vi "Write TDMS.vi"(8 "error in":errorcluster, 11 "Control Loop Cluster":T1) -> (0 "error out":errorcluster, 3 "Control Loop Cluster Out":T1)   [LabVIEW 2019, in "RT Main.lvlib"]
uses:
  RT Main.lvlib
  Control Loop Cluster.ctl
  <vilib>/myRIO/Instrument Drivers/Onboard IO/AI/typedefs/AI Reference.ctl
  <vilib>/myRIO/Common/Instrument Driver Framework/Utilities/typedefs/myRIO Generic Hardware Reference.ctl
  <vilib>/myRIO/Common/Instrument Driver Framework/Utilities/typedefs/Hardware Version Enum.ctl
  <vilib>/myRIO/Common/Instrument Driver Framework/Utilities/typedefs/myRIO v1.0 Reference.ctl
  <vilib>/myRIO/Common/Instrument Driver Framework/Utilities/typedefs/Generic FPGA Reference.ctl
  <vilib>/myRIO/Common/Instrument Driver Framework/myRIO v1.0/AI/typedefs/AI Channels List.ctl
  <vilib>/myRIO/Common/Instrument Driver Framework/myRIO v1.0/AI/typedefs/AI Channels Enum.ctl
  <vilib>/myRIO/Common/Instrument Driver Framework/Utilities/typedefs/Analog Scaling Constants List.ctl
  <vilib>/myRIO/Common/Instrument Driver Framework/Utilities/typedefs/Analog Scaling Constants.ctl
  <vilib>/myRIO/Instrument Drivers/Onboard IO/DIO/typedefs/DIO Reference.ctl
  <vilib>/myRIO/Common/Instrument Driver Framework/myRIO v1.0/DIO/typedefs/DIO Channels List.ctl
  <vilib>/myRIO/Common/Instrument Driver Framework/myRIO v1.0/DIO/typedefs/DIO Channels Enum.ctl
  Data Cluster.ctl
  Hardware Monitoring.ctl
  Modules/TDMS/TDMS.lvlib
  <vilib>/myRIO/Instrument Drivers/Onboard IO/AI/AI.lvlib
  <vilib>/myRIO/Instrument Drivers/Onboard IO/DIO/DIO.lvlib
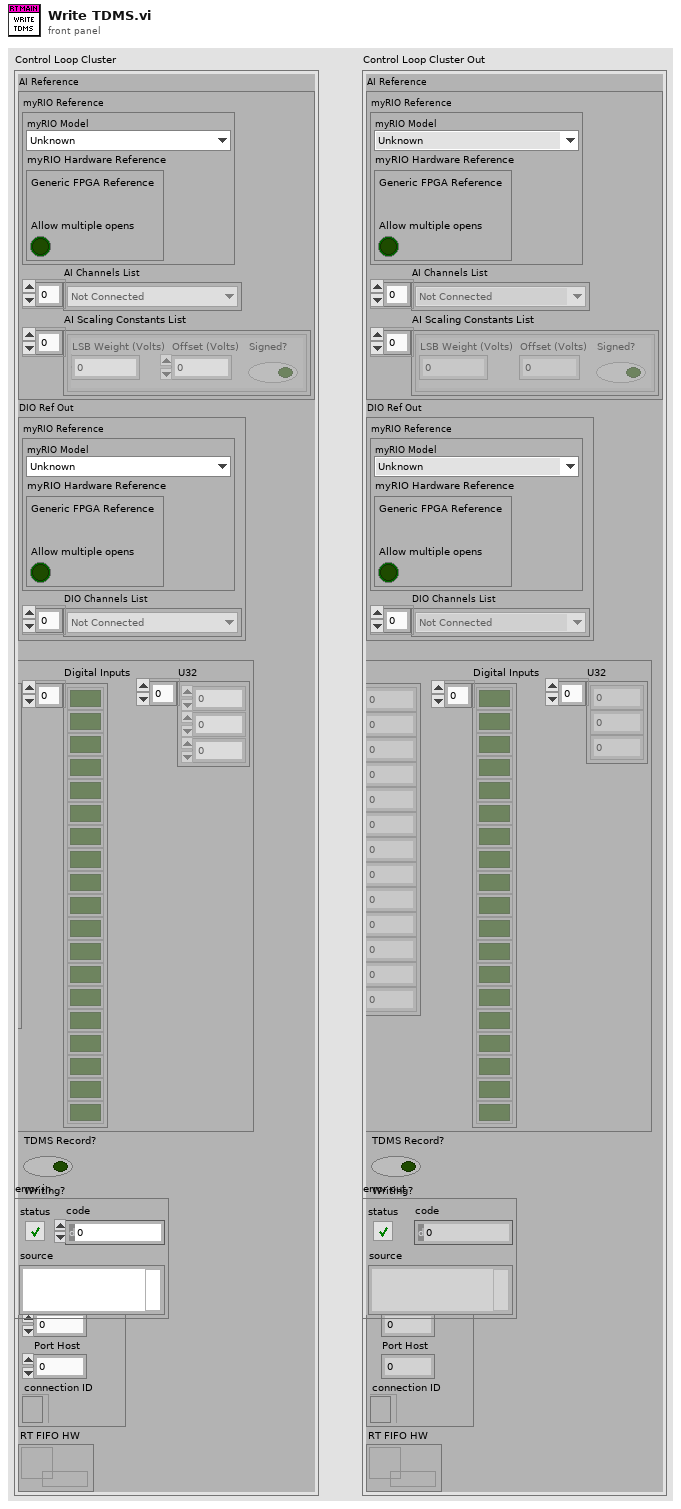
[diagram p1: front panel]
types:
  T1 = typedef "RT Main.lvlib/Control Loop Cluster.ctl" = cluster{"AI Reference":T2, "DIO Reference":T11, "Data Cluster":T14, "TDMS Record?":bool, "Writing?":bool, "UDP Info":cluster{"IP Host":string, "Port RT":u16, "Port Host":u16, "connection ID":refnum<k16>}, "RT FIFO HW":refnum<k33>}
  T2 = typedef "AI.lvlib/AI Reference.ctl" = cluster{"myRIO Reference":T3, "AI Channels List":T7, "AI Scaling Constants List":T9}
  T3 = typedef "myRIO Generic Hardware Reference.ctl" = cluster{"myRIO Model":T4, "myRIO Hardware Reference":T5}
  T4 = typedef "Hardware Version Enum.ctl" = enum16{"Unknown", "myRIO-1900", "myRIO-1950", "roboRIO", "NI ELVIS RIO CM", "ELVIS III"}
  T5 = typedef "myRIO v1.0 Reference.ctl" = cluster{"Generic FPGA Reference":T6, "Allow multiple opens":bool}
  T6 = typedef "Generic FPGA Reference.ctl" = refnum<k20>
  T7 = typedef "AI Channels List.ctl" = T8[]
  T8 = typedef "AI Channels Enum.ctl" = enum16{"Not Connected", "AudioIn/Left", "AudioIn/Right", "C/AI0", "C/AI1", "A/AI0", "A/AI1", "A/AI2", "A/AI3", "A/AI4", "A/AI5", "A/AI6", "A/AI7", "B/AI0", "B/AI1", "B/AI2", "B/AI3", "B/AI4", "B/AI5", "B/AI6", "B/AI7", "AI/AI0", "AI/AI1", "AI/AI2", "AI/AI3", "A/AI0 (DIFF)", "A/AI1 (DIFF)", "A/AI2 (DIFF)", "A/AI3 (DIFF)", "B/AI0 (DIFF)", "B/AI1 (DIFF)", "B/AI2 (DIFF)", "B/AI3 (DIFF)"}
  T9 = typedef "Analog Scaling Constants List.ctl" = T10[]
  T10 = typedef "Analog Scaling Constants.ctl" = cluster{"LSB Weight (Volts)":dbl, "Offset (Volts)":dbl, "Signed?":bool}
  T11 = typedef "DIO.lvlib/DIO Reference.ctl" = cluster{"myRIO Reference":T3, "DIO Channels List":T12}
  T12 = typedef "DIO Channels List.ctl" = T13[]
  T13 = typedef "DIO Channels Enum.ctl" = enum16{"Not Connected", "C/DIO0", "C/DIO1", "C/DIO2", "C/DIO3", "C/DIO4", "C/DIO5", "C/DIO6", "C/DIO7", "A/DIO0", "A/DIO1", "A/DIO2", "A/DIO3", "A/DIO4", "A/DIO5", "A/DIO6", "A/DIO7", "A/DIO8", "A/DIO9", "A/DIO10", "A/DIO11", "A/DIO12", "A/DIO13", "A/DIO14", "A/DIO15", "A/DIO16", "A/DIO17", "A/DIO18", "A/DIO19", "B/DIO0", "B/DIO1", "B/DIO2", "B/DIO3", "B/DIO4", "B/DIO5", "B/DIO6", "B/DIO7", "B/DIO8", "B/DIO9", "B/DIO10", "B/DIO11", "B/DIO12", "B/DIO13", "B/DIO14", "B/DIO15", "B/DIO16", "B/DIO17", "B/DIO18", "B/DIO19", "LED0", "LED1", "LED2", "LED3", "Button0", "DIO/DIO0", "DIO/DIO1", "DIO/DIO2", "DIO/DIO3", "DIO/DIO4", "DIO/DIO5", "DIO/DIO6", "DIO/DIO7", "DIO/DIO8", "DIO/DIO9", "SPI/CS0", "SPI/CS1", "SPI/CS2", "SPI/CS3", "LED RADIO (Green)", "LED RADIO (Red)", "LED COMM (Green)", "LED COMM (Red)", "LED MODE (Green)", "LED MODE (Red)"}
  T14 = typedef "RT Main.lvlib/Data Cluster.ctl" = cluster{"Analog Input":dbl[], "Digital Inputs":bool[], "U32":u32[]}
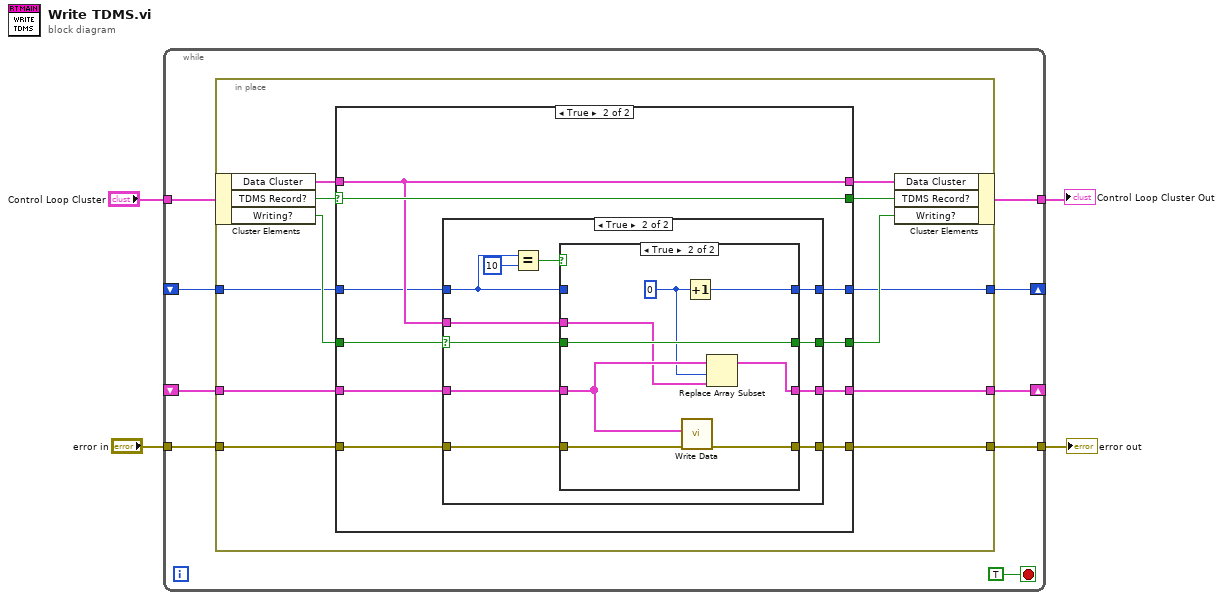
[diagram p0: block diagram]
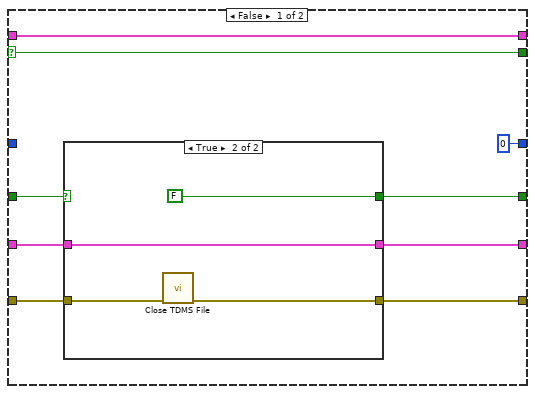
[diagram p2: hidden frame]
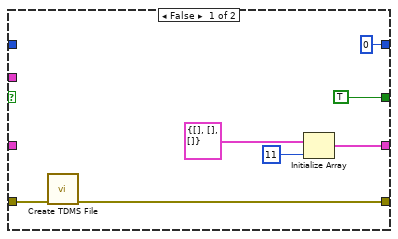
[diagram p4: hidden frame]
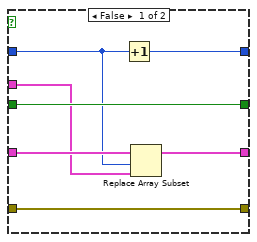
[diagram p5: hidden frame]
diagram:
  n1 = while {
    tunnel: "Control Loop Cluster" -> [w13]
    tunnel: "error in" -> [w12]
    tunnel: [w11] -> w2
    tunnel: [w9] -> w1
    shift-right: [w8] -> _
    shift-left: _ -> [w7]
    shift-right: [w6] -> _
    shift-left: _ -> [w5]
    stop <- TRUE stop-if-true
    n2 = in-place {
      in-place-border: w12 -> [w21]
      in-place-border: [w20] -> w9
      in-place-border: [w19] -> w8
      in-place-border: w7 -> [w18]
      in-place-border: [w15] -> w6
      in-place-border: w5 -> [w14]
      n3 = in-place-cluster #1(w13) -> ("Data Cluster"=w22:T14, "TDMS Record?"=w25:bool, "Writing?"=w17:bool)
      n4 = case shown="True" w25 {
        selector: w25 -> [w34 w51]
        tunnel: [w34 w51] -> w24
        tunnel: [w33 w46] -> w23
        tunnel: w22 -> [w33 w46]
        tunnel: [w31 w50] -> w16
        tunnel: w17 -> [w32 w49]
        tunnel: w21 -> [w30 w48]
        tunnel: [w29 w47] -> w20
        tunnel: [w27 w45] -> w19
        tunnel: w18 -> [w26 w44]
        tunnel: [0 w43] -> w15
        tunnel: w14 -> [_ w42]
        frame False {
          n5 = case shown="True" w32 {
            selector: w32 -> [w37 _]
            tunnel: [w37 FALSE] -> w31
            tunnel: w30 -> [w36 w40]
            tunnel: [w36 w39] -> w29
            tunnel: [w35 w38] -> w27
            tunnel: w26 -> [w35 w38]
            frame False {
            }
            frame True {
              n6 = call "Close TDMS File.vi"("error in"=w40) -> ("error out"=w39:errorcluster)  [unwired: 10 in]
            }
          }
        }
        frame True {
          n7 = case shown="True" w49 {
            selector: w49 -> [_ w68]
            tunnel: [TRUE w69] -> w50
            tunnel: w48 -> [w57 w67]
            tunnel: [w56 w66] -> w47
            tunnel: w46 -> [_ w65]
            tunnel: [w54 w63] -> w45
            tunnel: w44 -> [_ w64]
            tunnel: [0 w62] -> w43
            tunnel: w42 -> [_ w59]
            frame False {
              n8 = call "Create TDMS File.vi"("error in"=w57) -> ("error out"=w56:errorcluster)  [unwired: 10 in]
              n9 = Initialize Array(T14 {"Analog Input"=[], "Digital Inputs"=[], "U32"=[]} ("Data Cluster"), 11 ("dimension size")) -> (w54:T14[])
            }
            frame True {
              n10 = Equal?(x=w59, y=10) -> (x = y?=w61:bool)
              n11 = case shown="True" w61 {
                tunnel: [w76 w84] -> w69
                tunnel: w68 -> [w76 w84]
                tunnel: w67 -> [w75 w83]
                tunnel: [w75 w82] -> w66
                tunnel: w65 -> [w70 w79]
                tunnel: w64 -> [w74 w80]
                tunnel: [w73 w77] -> w63
                tunnel: [w71 w81] -> w62
                tunnel: w59 -> [w72 _]
                frame False {
                  n12 = Increment(x=w72) -> (x+1=w71:i32)
                  n13 = Replace Array Subset "Replace Array Subset"(array=w74, new element=w70, index=w72) -> (w73:T14[])
                }
                frame True {
                  w78 = 0
                  n14 = call "Write Data.vi"("error in"=w83, "array"=w80) -> ("error out"=w82:errorcluster)  [unwired: 9 in]
                  n15 = Increment(x=w78) -> (x+1=w81:i32)
                  n16 = Replace Array Subset(array=w80, new element=w79, index=w78) -> (w77:T14[])
                }
              }
            }
          }
        }
      }
      n17 = in-place-cluster #1("Data Cluster"=w23, "TDMS Record?"=w24, "Writing?"=w16) -> (w11:T1)
    }
  }
  "Control Loop Cluster Out" <- w2
  "error out" <- w1
